vi "Open.vi"(4 "Delimiter":string=",", 6 "File Extension":string="csv", 7 "Start Time Stamp":timestamp, 8 "Error In":errorcluster, 10 "Enable Calendar Tree":bool=TRUE, 11 "Base Folder":path) -> (0 "Error Out":errorcluster, 3 "Log Out":refnum<file>)   [LabVIEW 2025, in "LOGlib_LV2025.lvlib" / "File.lvlib"]
uses:
  File.lvlib
  <vilib>/Utility/libraryn.llb/Check if File or Folder Exists.vi
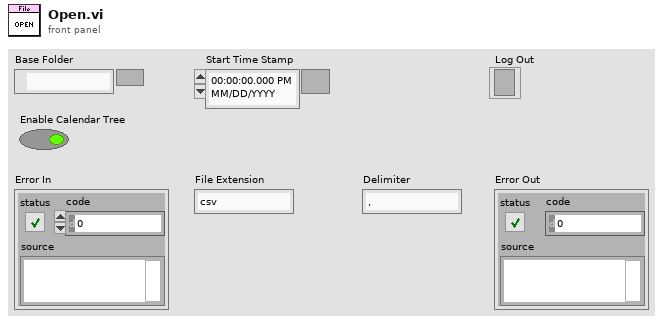
[diagram p1: front panel]
types:
  T1 = enum16{"open", "replace", "create", "open or create", "replace or create", "replace or create with confirmation"}
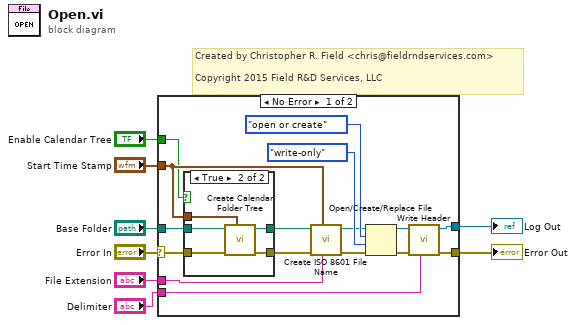
[diagram p0: block diagram]
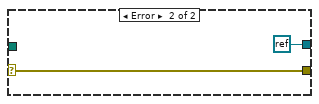
[diagram p3: hidden frame]
diagram:
  # "Created by Christopher R. Field <chris@fieldrndservices.com>\n\nCopyright 2015 Field R&D Services, LLC"
  n1 = case shown="No Error" "Error In" {
    selector: "Error In" -> [w21 w33]
    tunnel: "Base Folder" -> [w22 _]
    tunnel: "Start Time Stamp" -> [w18 _]
    tunnel: [w12 refnum<k0> refnum] -> w5
    tunnel: [w11 w33] -> w4
    tunnel: "Enable Calendar Tree" -> [w13 _]
    tunnel: "File Extension" -> [w10 _]
    tunnel: "Delimiter" -> [w9 _]
    frame No Error {
      n2 = case shown="True" w13 {
        tunnel: w22 -> [w26 w31]
        tunnel: w21 -> [w25 w30]
        tunnel: [w26 w29] -> w20
        tunnel: [w25 w28] -> w19
        tunnel: w18 -> [_ w27]
        frame False {
        }
        frame True {
          n3 = call "Create Calendar Folder Tree.vi"("Start Time Stamp"=w27, "Error In"=w30, "Base Log Folder"=w31) -> ("Error Out"=w28:errorcluster, "Calendar Folder Tree"=w29:path)  [unwired: 7 in]
        }
      }
      n4 = call "Create ISO 8601 File Name.vi"("File Extension"=w10, "Start Time Stamp"=w18, "Error In"=w19, "Log Folder"=w20) -> ("Error Out"=w16:errorcluster, "ISO 8601 File"=w17:path)  [unwired: 6 in]
      n5 = Open/Create/Replace File(file path (use dialog)=w17, error in=w16, operation (0:open)=T1."open or create", access (0:read/write)=enum16{"read/write", "read-only", "write-only"}."write-only") -> (refnum out=w15:refnum<file>, error out=w14:errorcluster)  [unwired: 2 in, 1 out]
      n6 = call "Write Header.vi"("Delimiter"=w9, "Error In"=w14, "Log In"=w15) -> ("Error Out"=w11:errorcluster, "Log Out"=w12:refnum<file>)  [unwired: 7 in]
    }
    frame Error {
    }
  }
  "Log Out" <- w5
  "Error Out" <- w4
